vi "Get Signal Direction.vi"(8 "error in (no error)":errorcluster, 11 "IO Class in":refnum<class "Signal.lvclass">) -> (0 "error out":errorcluster, 2 "Direction":enum16{"Input", "Output", "Unused"}(ring), 3 "IO Class out":refnum<class "Signal.lvclass">)   [LabVIEW 2025, in "Signal.lvclass"]
doc: "Get the signal direction (input, output, our unused)"
uses:
  Signal.lvclass
  Configuration.ctl
  Read Configuration.vi
  <vilib>/Utility/Data Type/NI_Data Type.lvlib
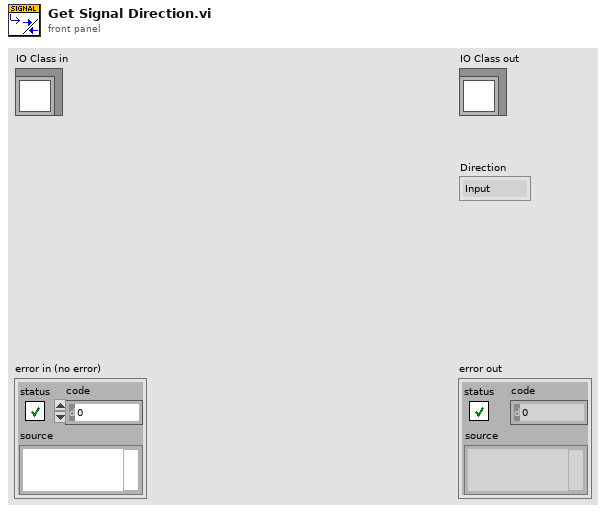
[diagram p1: front panel]
types:
  T1 = typedef "Signal.lvclass/Configuration.ctl" = cluster{"Classification":string, "Direction":string, "Type":string}
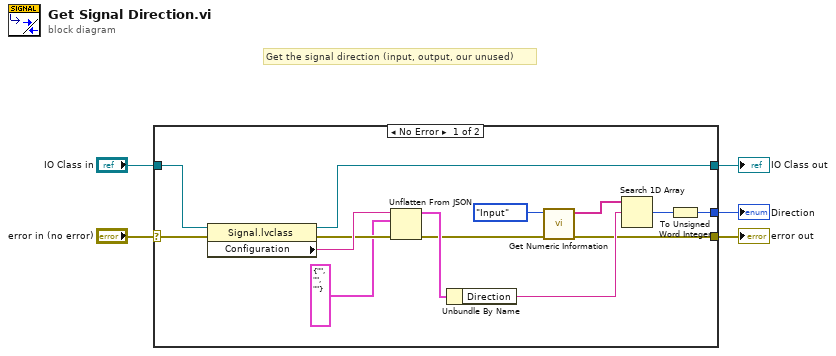
[diagram p0: block diagram]
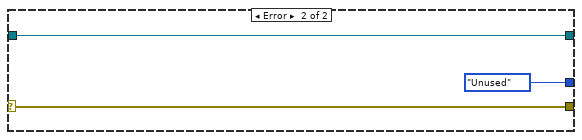
[diagram p2: hidden frame]
diagram:
  # "Get the signal direction (input, output, our unused)"
  n1 = case shown="No Error" "error in (no error)" {
    selector: "error in (no error)" -> [w15 w22]
    tunnel: [w6 w22] -> w4
    tunnel: [w13 w21] -> w2
    tunnel: "IO Class in" -> [w14 w21]
    tunnel: [w7 enum16{"Input", "Output", "Unused"}."Unused" ("Direction")] -> w1
    frame No Error {
      n2 = property class="Signal.lvclass"(reference=w14, error in=w15) -> (reference out=w13:refnum<class "Signal.lvclass">, error out=w18:errorcluster, "Configuration"=w19:string)
      n3 = Unflatten From JSON(JSON string=w19, type and defaults=T1 {"Classification"="", "Direction"="", "Type"=""} ("Configuration"), error in (no error)=w18) -> (value=w17:T1, error out=w9:errorcluster)  [unwired: 4 in]
      n4 = Unbundle By Name(w17) -> ("Direction"=w8:string)
      n5 = call <vilib>:"Get Numeric Information.vi"("error in (no error)"=w9, "variant"=enum16{"Input", "Output", "Unused"}."Input" ("Direction")) -> ("error out"=w6:errorcluster, "enum names"=w12:string[])  [unwired: 6 in, 2 out]
      n6 = Search 1D Array(1D array=w12, element=w8) -> (index of element=w11:i32)  [unwired: 1 in]
      n7 = To Unsigned Word Integer(number=w11) -> (unsigned 16bit integer=w7:u16)
    }
    frame Error {
    }
  }
  "error out" <- w4
  "IO Class out" <- w2
  "Direction" <- w1
